vi "Check Parameters.vi"(0 "ToneCloud in":refnum<class "Tone Cloud.lvclass">, 9 "Fs (Hz)":dbl, 11 "error in (no error)":errorcluster) -> (4 "ToneCloud out":refnum<class "Tone Cloud.lvclass">, 15 "error out":errorcluster)   [LabVIEW 2015, in "Tone Cloud.lvclass"]
uses:
  Tone Cloud.lvclass
  Tone Cloud.lvclass/Tone Cloud.ctl
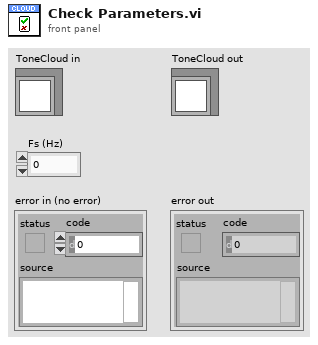
[diagram p1: front panel]
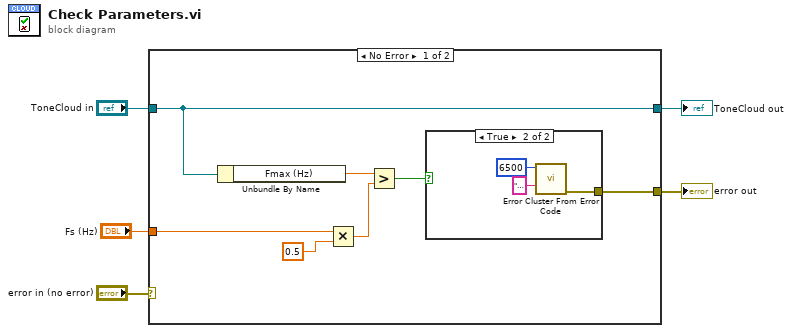
[diagram p0: block diagram]
diagram:
  n1 = case shown="No Error" "error in (no error)" {
    selector: "error in (no error)" -> [_ w17]
    tunnel: [w6 w17] -> w4
    tunnel: [w12 w16] -> w2
    tunnel: "ToneCloud in" -> [w12 w16]
    tunnel: "Fs (Hz)" -> [w9 _]
    frame No Error {
      n2 = Unbundle By Name(w12) -> ("Fmax (Hz)"=w8:dbl)
      n3 = Multiply(x=w9, y=0.5) -> (x*y=w11:dbl)
      n4 = Greater?(x=w8, y=w11) -> (0:w7:bool)
      n5 = case shown="True" w7 {
        tunnel: [_ w14] -> w6
        frame False {
        }
        frame True {
          n6 = call <vilib>:"Error Cluster From Error Code.vi"("error message (\"\")"="Tone Cloud: Fmax exceeds the Nyquist frequency. Increase the sampling rate or decrease Fmax." ("error message (\"\")"), "error code (0)"=6500) -> ("error out"=w14:errorcluster)  [unwired: 7 in]
        }
      }
    }
    frame Error {
    }
  }
  "error out" <- w4
  "ToneCloud out" <- w2
